vi "Parse Numeric.vi"(0 "JSON String":string, 5 "Index In":i32, 11 "error in (no error)":errorcluster) -> (4 "Variant out":variant, 6 "Index Out":i32, 15 "error out":errorcluster)   [LabVIEW 2020, in "Variant JSON API.lvlib"]
uses:
  Variant JSON API.lvlib
  Errors.ctl
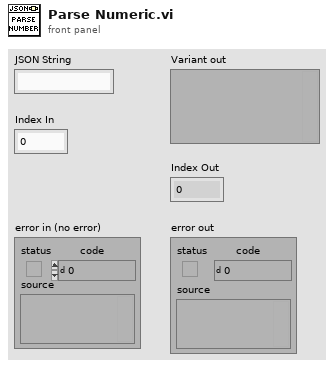
[diagram p1: front panel]
types:
  T1 = typedef "Variant JSON API.lvlib/Errors.ctl" = enum16{"No key", "Key path type", "Array OOB", "Type Mismatch", "Invalid Token", "Invalid Value"}
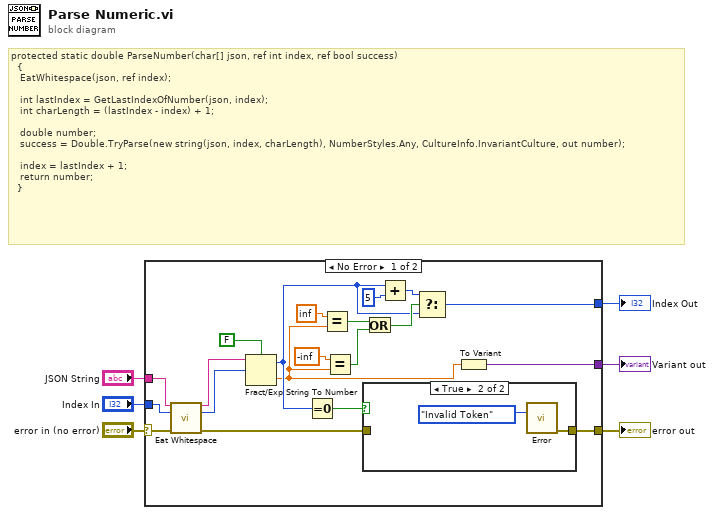
[diagram p0: block diagram]
diagram:
  # "protected static double ParseNumber(char[] json, ref int index, ref bool success)\n\t\t{\n\t\t\tEatWhitespace(json, ref index);\n\n\t\t\tint lastIndex = GetLastIndexOfNumber(json, index);\n\t\t\tint charLength = (lastIndex - index) + 1;\n\n\t\t\tdouble number;\n\t\t\tsuccess = Double.TryParse(new string(json, index, charLength), NumberStyles.Any, CultureInfo.InvariantCulture, out number);\n\n\t\t\tindex = lastIndex + 1;\n\t\t\treturn number;\n\t\t}"
  n1 = case shown="No Error" "error in (no error)" {
    selector: "error in (no error)" -> [w25 w30]
    tunnel: [w9 w30] -> w5
    tunnel: [w7 _] -> w1
    tunnel: "Index In" -> [w26 w31]
    tunnel: [w10 w31] -> w3
    tunnel: "JSON String" -> [w19 _]
    frame No Error {
      n2 = call "Eat Whitespace.vi"("JSON String"=w19, "Index In"=w26, "error in (no error)"=w25) -> ("JSON String Passthrough"=w24:string, "Index Out"=w23:i32, "error out"=w21:errorcluster)  [unwired: 10 in]
      n3 = Fract/Exp String To Number(use system decimal point (T)=FALSE, string=w24, offset=w23) -> (offset past number=w13:i32, number=w8:dbl)  [unwired: 1 in]
      n4 = Equal To 0?(x=w13) -> (x = 0?=w22:bool)
      n5 = Equal?(x=inf, y=w8) -> (x = y?=w17:bool)
      n6 = Equal?(x=-inf, y=w8) -> (x = y?=w15:bool)
      n7 = case shown="True" w22 {
        tunnel: w21 -> [w27 _]
        tunnel: [w27 w29] -> w9
        frame False {
        }
        frame True {
          n8 = call "Error.vi"(5:Errors."Invalid Token") -> ("error out"=w29:errorcluster)  [unwired: 14 in]
        }
      }
      n9 = Or(x=w17, y=w15) -> (x .or. y?=w14:bool)
      n10 = Add(x=w13, y=5) -> (x+y=w11:i32)
      n11 = Select(t=w11, s=w14, f=w13) -> (s? t:f=w10:i32)
      n12 = To Variant(anything=w8) -> (Variant=w7:variant)
    }
    frame Error {
    }
  }
  "error out" <- w5
  "Index Out" <- w3
  "Variant out" <- w1
